vi "APC_rpm_to_4_20mA.vi"(1 "Perc0_100":dbl format="%.2f") -> (0 "fixed-point":fxp<+,20,-5> format="%#_7g")   [LabVIEW 2020]
panel:
  out "x+y":dbl
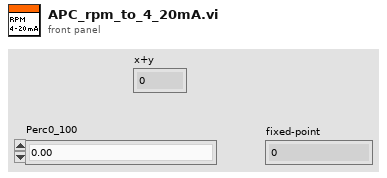
[diagram p1: front panel]
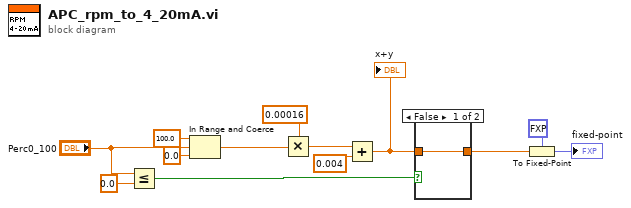
[diagram p0: block diagram]
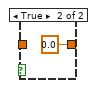
[diagram p2: hidden frame]
diagram:
  n1 = Less Or Equal?(x="Perc0_100", y=0.0) -> (x <= y?=w5:bool)
  n2 = In Range and Coerce(upper limit=100.0, x="Perc0_100", lower limit=0.0) -> (coerced(x)=w3:dbl)  [unwired: 1 out]
  n3 = Multiply(x=0.00016, y=w3) -> (x*y=w12:dbl)
  n4 = Add(x=w12, y=0.004) -> (x+y=w8:dbl)
  "x+y" <- w8
  n5 = case shown="False" w5 {
    tunnel: w8 -> [w14 _]
    tunnel: [w14 0.0] -> w7
    frame False {
    }
    frame True {
    }
  }
  n6 = To Fixed-Point(fixed-point type=fxp<+,20,-5> 0.0 ("NI9266/AO7"), number=w7) -> (fixed-point=→"fixed-point":fxp<+,20,-5>)
